vi "Update.vi"(8 "error in (no error)":errorcluster, 10 "Message in":refnum<class "UpdateMessage.lvclass">, 11 "Tomo in":refnum<class "Tomo.lvclass">) -> (0 "error out":errorcluster, 3 "Tomo out":refnum<class "Tomo.lvclass">)   [LabVIEW 2012, in "Tomo.lvclass"]
doc: "The update method processes the command 'update'. \n\nThe command 'update' is used for receiving new values to be set to the private data of the class. This could be seen as a public set method for setting new parameters to the private class data."
uses:
  Tomo.lvclass
  <vilib>/Distrio/Murmex/UpdateMessage/UpdateMessage.lvclass
  Tomo.lvclass/Tomo.ctl
  <vilib>/Distrio/Murmex/GenericMessage/GenericMessage.lvclass
  <vilib>/Distrio/Murmex/Murmex/Murmex.lvclass
  <vilib>/Distrio/Murmex/Message/Add or replace parameter.vi
panel:
  # "This method is called when the UPDATE\ntrigger is sent. \n\nOverride this method when your component needs to\nrespond to this trigger. \n\nCall parent for proper implementation"
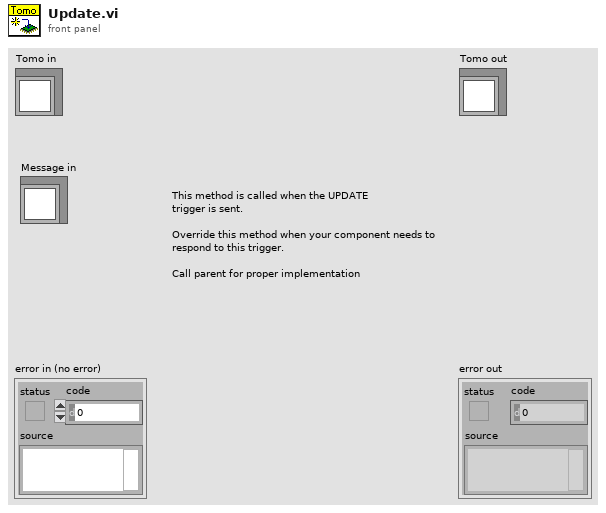
[diagram p1: front panel]
types:
  T1 = enum16{"Cubic volume", "Custom volume", "Self-generate volume"}
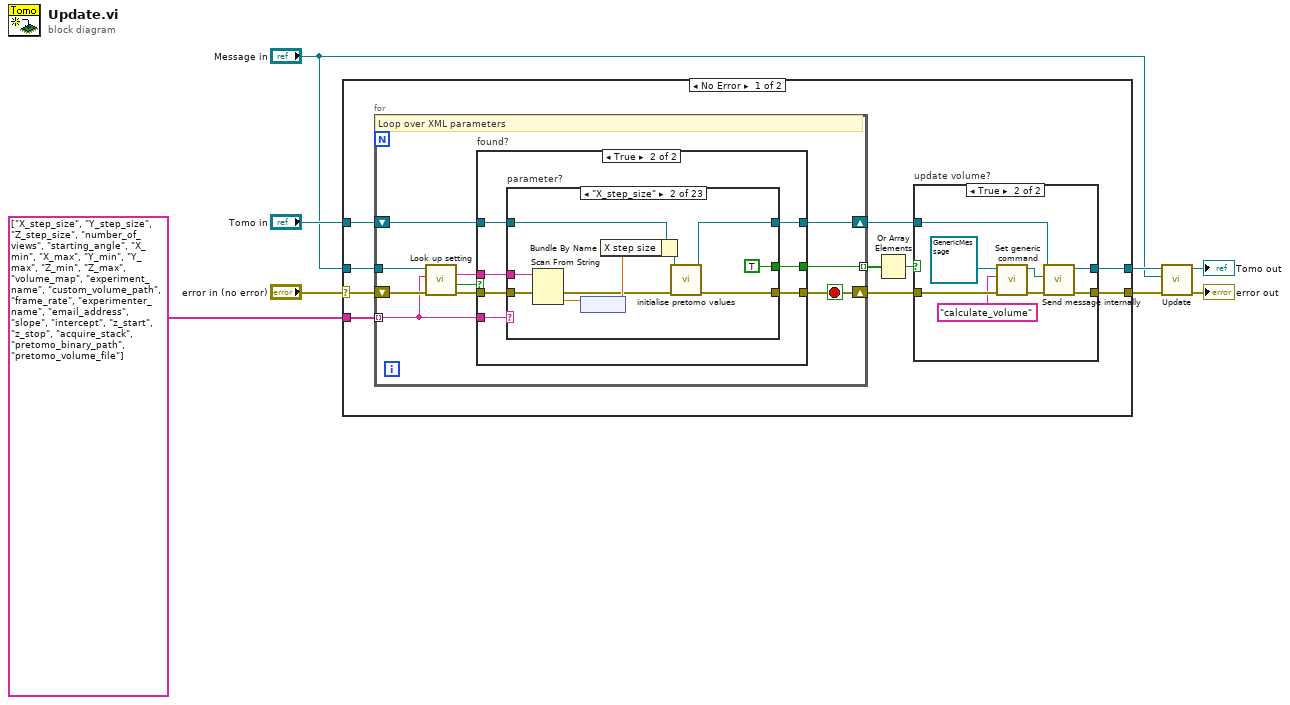
[diagram p0: block diagram]
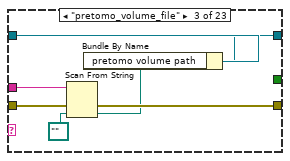
[diagram p5: hidden frame]
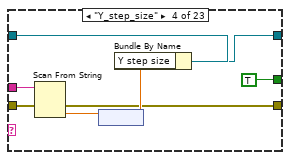
[diagram p6: hidden frame]
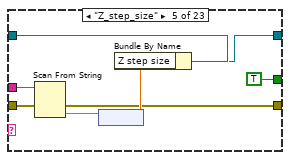
[diagram p7: hidden frame]
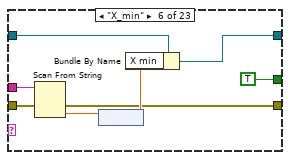
[diagram p8: hidden frame]
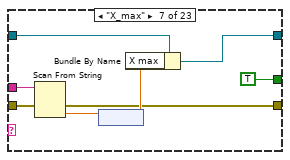
[diagram p9: hidden frame]
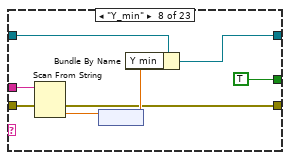
[diagram p10: hidden frame]
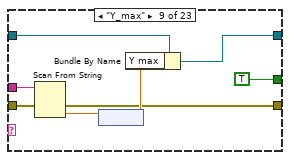
[diagram p11: hidden frame]
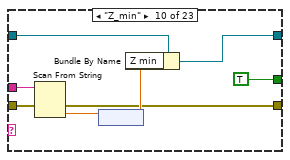
[diagram p12: hidden frame]
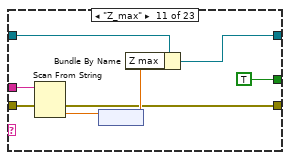
[diagram p13: hidden frame]
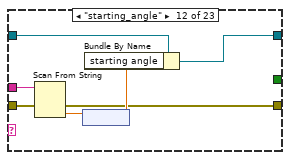
[diagram p14: hidden frame]
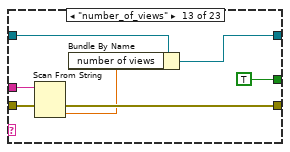
[diagram p15: hidden frame]
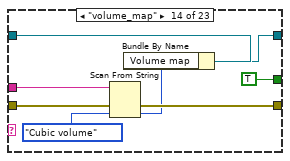
[diagram p16: hidden frame]
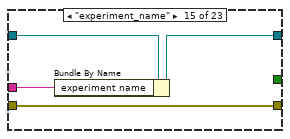
[diagram p17: hidden frame]
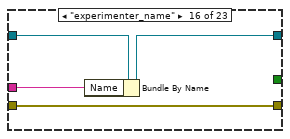
[diagram p18: hidden frame]
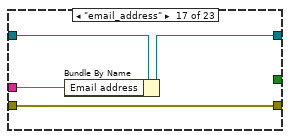
[diagram p19: hidden frame]
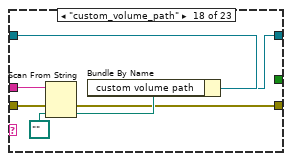
[diagram p20: hidden frame]
diagram:
  n1 = case shown="No Error" "error in (no error)" {
    selector: "error in (no error)" -> [w18 w208]
    tunnel: "Message in" -> [w17 _]
    tunnel: "Tomo in" -> [w16 w209]
    tunnel: string[] ["X_step_size", "Y_step_size", "Z_step_size", "number_of_views", "starting_angle", "X_min", "X_max", "Y_min", "Y_max", "Z_min", "Z_max", "volume_map", "experiment_name", "custom_volume_path", "frame_rate", "experimenter_name", "email_address", "slope", "intercept", "z_start", "z_stop", "acquire_stack", "pretomo_binary_path", "pretomo_volume_file"] -> [w15 _]
    tunnel: [w13 w208] -> w3
    tunnel: [w11 w209] -> w2
    frame No Error {
      n2 = for {
        shift-right: [w31] -> w14
        shift-left: w18 -> [w38]
        tunnel: w17 -> [w37]
        shift-right: [w32] -> w12
        shift-left: w16 -> [w33]
        tunnel: w15 -> [w30] mode=indexing
        tunnel: [w29] -> w10 mode=indexing
        stop <- w31 stop-if-true
        # "Loop over XML parameters"
        n3 = call <vilib>:"Look up setting.vi"("error in (no error)"=w38, "tag name"=w30, "UpdateMessage in"=w37) -> ("error out"=w35:errorcluster, "found?"=w36:bool, "value"=w34:string)  [unwired: 5 in, 1 out]
        n4 = case "found?" shown="True" w36 {
          tunnel: w30 -> [_ w47]
          tunnel: w35 -> [w39 w45]
          tunnel: w34 -> [_ w44]
          tunnel: w33 -> [w40 w46]
          tunnel: [w39 w43] -> w31
          tunnel: [w40 w42] -> w32
          tunnel: [_ w41] -> w29
          frame False {
          }
          frame True {
            n5 = case "parameter?" shown="\"X_step_size\"" w47 {
              tunnel: w46 -> [w49 w57 w64 w72 w80 w88 w96 w104 w112 w120 w128 w135 w142 w150 w156 w160 w164 w171 w179 w184 w191 w198 w205]
              tunnel: w45 -> [w48 w59 w66 w74 w82 w90 w98 w106 w114 w122 w130 w137 w144 w152 w154 w158 w162 w165 w174 w186 w193 w200 w207]
              tunnel: w44 -> [_ w58 w65 w73 w81 w89 w97 w105 w113 w121 w129 w136 w143 w151 w153 w157 w161 w169 w177 w180 w187 w194 w202]
              tunnel: [w48 w52 w63 w69 w77 w85 w93 w101 w109 w117 w125 w132 w141 w149 w154 w158 w162 w166 w175 w185 w192 w199 w206] -> w43
              tunnel: [w49 w50 w62 w68 w76 w84 w92 w100 w108 w116 w124 w131 w140 w148 w155 w159 w163 w170 w178 w183 w190 w197 w204] -> w42
              tunnel: [_ TRUE _ TRUE TRUE TRUE TRUE TRUE TRUE TRUE TRUE _ TRUE TRUE _ _ _ _ TRUE _ _ _ _] -> w41
              frame Default {
              }
              frame "X_step_size" {
                n6 = Scan From String(input string=w58, error in=w59) -> (error out=w53:errorcluster, output 1=w55:dbl)  [unwired: 3 in, 2 out]
                n7 = node(w55) -> (w56:dbl[unit])
                n8 = Bundle By Name(cluster=w57, "X step size"=w56) -> (w51:refnum<class "Tomo.lvclass">)
                n9 = call-dynamic "initialise pretomo values.vi"("error in (no error)"=w53, "Tomo in"=w51) -> ("error out"=w52:errorcluster, "Tomo out"=w50:refnum<class "Tomo.lvclass">)  [unwired: 8 in]
              }
              frame "pretomo_volume_file" {
                n10 = Scan From String(input string=w65, error in=w66, default 1=path "") -> (error out=w63:errorcluster, output 1=w60:path)  [unwired: 2 in, 2 out]
                n11 = Bundle By Name(cluster=w64, "pretomo volume path"=w60) -> (w62:refnum<class "Tomo.lvclass">)
              }
              frame "Y_step_size" {
                n12 = Scan From String(input string=w73, error in=w74) -> (error out=w69:errorcluster, output 1=w70:dbl)  [unwired: 3 in, 2 out]
                n13 = node(w70) -> (w71:dbl[unit])
                n14 = Bundle By Name(cluster=w72, "Y step size"=w71) -> (w68:refnum<class "Tomo.lvclass">)
              }
              frame "Z_step_size" {
                n15 = Scan From String(input string=w81, error in=w82) -> (error out=w77:errorcluster, output 1=w78:dbl)  [unwired: 3 in, 2 out]
                n16 = node(w78) -> (w79:dbl[unit])
                n17 = Bundle By Name(cluster=w80, "Z step size"=w79) -> (w76:refnum<class "Tomo.lvclass">)
              }
              frame "X_min" {
                n18 = Scan From String(input string=w89, error in=w90) -> (error out=w85:errorcluster, output 1=w86:dbl)  [unwired: 3 in, 2 out]
                n19 = node(w86) -> (w87:dbl[unit])
                n20 = Bundle By Name(cluster=w88, "X min"=w87) -> (w84:refnum<class "Tomo.lvclass">)
              }
              frame "X_max" {
                n21 = Scan From String(input string=w97, error in=w98) -> (error out=w93:errorcluster, output 1=w94:dbl)  [unwired: 3 in, 2 out]
                n22 = node(w94) -> (w95:dbl[unit])
                n23 = Bundle By Name(cluster=w96, "X max"=w95) -> (w92:refnum<class "Tomo.lvclass">)
              }
              frame "Y_min" {
                n24 = Scan From String(input string=w105, error in=w106) -> (error out=w101:errorcluster, output 1=w102:dbl)  [unwired: 3 in, 2 out]
                n25 = node(w102) -> (w103:dbl[unit])
                n26 = Bundle By Name(cluster=w104, "Y min"=w103) -> (w100:refnum<class "Tomo.lvclass">)
              }
              frame "Y_max" {
                n27 = Scan From String(input string=w113, error in=w114) -> (error out=w109:errorcluster, output 1=w110:dbl)  [unwired: 3 in, 2 out]
                n28 = node(w110) -> (w111:dbl[unit])
                n29 = Bundle By Name(cluster=w112, "Y max"=w111) -> (w108:refnum<class "Tomo.lvclass">)
              }
              frame "Z_min" {
                n30 = Scan From String(input string=w121, error in=w122) -> (error out=w117:errorcluster, output 1=w118:dbl)  [unwired: 3 in, 2 out]
                n31 = node(w118) -> (w119:dbl[unit])
                n32 = Bundle By Name(cluster=w120, "Z min"=w119) -> (w116:refnum<class "Tomo.lvclass">)
              }
              frame "Z_max" {
                n33 = Scan From String(input string=w129, error in=w130) -> (error out=w125:errorcluster, output 1=w126:dbl)  [unwired: 3 in, 2 out]
                n34 = node(w126) -> (w127:dbl[unit])
                n35 = Bundle By Name(cluster=w128, "Z max"=w127) -> (w124:refnum<class "Tomo.lvclass">)
              }
              frame "starting_angle" {
                n36 = Scan From String(input string=w136, error in=w137) -> (error out=w132:errorcluster, output 1=w133:dbl)  [unwired: 3 in, 2 out]
                n37 = node(w133) -> (w134:dbl[unit])
                n38 = Bundle By Name(cluster=w135, "starting angle"=w134) -> (w131:refnum<class "Tomo.lvclass">)
              }
              frame "number_of_views" {
                n39 = Scan From String(input string=w143, error in=w144) -> (error out=w141:errorcluster, output 1=w139:dbl)  [unwired: 3 in, 2 out]
                n40 = Bundle By Name(cluster=w142, "number of views"=w139) -> (w140:refnum<class "Tomo.lvclass">)
              }
              frame "volume_map" {
                n41 = Scan From String(input string=w151, error in=w152, default 1=T1."Cubic volume" ("Volume map")) -> (error out=w149:errorcluster, output 1=w146:T1)  [unwired: 2 in, 2 out]
                n42 = Bundle By Name(cluster=w150, "Volume map"=w146) -> (w148:refnum<class "Tomo.lvclass">)
              }
              frame "experiment_name" {
                n43 = Bundle By Name(cluster=w156, "experiment name"=w153) -> (w155:refnum<class "Tomo.lvclass">)
              }
              frame "experimenter_name" {
                n44 = Bundle By Name(cluster=w160, "Name"=w157) -> (w159:refnum<class "Tomo.lvclass">)
              }
              frame "email_address" {
                n45 = Bundle By Name(cluster=w164, "Email address"=w161) -> (w163:refnum<class "Tomo.lvclass">)
              }
              frame "custom_volume_path" {
                n46 = Scan From String(input string=w169, error in=w165, default 1=path "") -> (error out=w166:errorcluster, output 1=w167:path)  [unwired: 2 in, 2 out]
                n47 = Bundle By Name(cluster=w171, "custom volume path"=w167) -> (w170:refnum<class "Tomo.lvclass">)
              }
              frame "frame_rate" {
                n48 = Scan From String(input string=w177, error in=w174) -> (error out=w175:errorcluster, output 1=w176:dbl)  [unwired: 3 in, 2 out]
                n49 = node(w176) -> (w173:dbl[unit])
                n50 = Bundle By Name(cluster=w179, "Frame rate"=w173) -> (w178:refnum<class "Tomo.lvclass">)
              }
              frame "z_start" {
                n51 = Scan From String(input string=w180, error in=w186) -> (error out=w185:errorcluster, output 1=w182:dbl)  [unwired: 3 in, 2 out]
                n52 = node(w182) -> (w181:dbl[unit])
                n53 = Bundle By Name(cluster=w184, "Z start"=w181) -> (w183:refnum<class "Tomo.lvclass">)
              }
              frame "z_stop" {
                n54 = Scan From String(input string=w187, error in=w193) -> (error out=w192:errorcluster, output 1=w189:dbl)  [unwired: 3 in, 2 out]
                n55 = node(w189) -> (w188:dbl[unit])
                n56 = Bundle By Name(cluster=w191, "Z stop"=w188) -> (w190:refnum<class "Tomo.lvclass">)
              }
              frame "acquire_stack" {
                n57 = Scan From String(input string=w194, error in=w200, default 1=TRUE) -> (error out=w199:errorcluster, output 1=w195:bool)  [unwired: 2 in, 2 out]
                n58 = Bundle By Name(cluster=w198, "above threshold?"=w195) -> (w197:refnum<class "Tomo.lvclass">)
              }
              frame "pretomo_binary_path" {
                n59 = Scan From String(input string=w202, error in=w207, default 1=path "") -> (error out=w206:errorcluster, output 1=w203:path)  [unwired: 2 in, 2 out]
                n60 = Bundle By Name(cluster=w205, "pretomo binary path"=w203) -> (w204:refnum<class "Tomo.lvclass">)
              }
            }
          }
        }
      }
      n61 = Or Array Elements(Boolean array=w10) -> (logical OR=w9:bool)
      n62 = case "update volume?" shown="True" w9 {
        tunnel: w14 -> [w19 w28]
        tunnel: [w19 w27] -> w13
        tunnel: w12 -> [w20 w25]
        tunnel: [w20 w24] -> w11
        frame False {
        }
        frame True {
          n63 = call <vilib>:"Set generic command.vi"("error in (no error)"=w28, "generic command"="calculate_volume", "GenericMessage in"=refnum<class "GenericMessage.lvclass"> refnum) -> ("error out"=w26:errorcluster, "GenericMessage out"=w23:refnum<class "GenericMessage.lvclass">)  [unwired: 7 in]
          n64 = call <vilib>:"Send message internally.vi"("error in (no error)"=w26, "Message"=w23, "Murmex in"=w25) -> ("error out"=w27:errorcluster, "Murmex out"=w24:refnum<class "Tomo.lvclass">)  [unwired: 7 in]
        }
      }
    }
    frame Error {
    }
  }
  n65 = call-parent "Update.vi"("error in (no error)"=w3, "Message in"="Message in", "Murmex in"=w2) -> ("error out"=→"error out":errorcluster, "Murmex out"=→"Tomo out":refnum<class "Tomo.lvclass">)  [unwired: 7 in]
